vi "Main.vi"() -> ()   [LabVIEW 2018]
doc: "This example sets the RS-485 transceiver control modes for the specified port and performs a serial port read, a serial port write, or a combination of these actions. If all are selected, the VI will write the data first, read data and then close the VISA session that is opened to the port. This VI will wait until the specified number of bytes is received at the port or until a termination character is received. This example will work only with National Instruments RS-485 interfaces.\n\nThis example demonstrates the transceiver control modes available when using a National Instruments RS-485 product. When connecting one or several devices via RS-485, a user may want to cut down on the amount of wiring. Alternatively, some devices offer a certain wiring configuration that you may need to match. Determine the wiring needs of the connected serial device to determine which NI RS-485 transceiver control mode to choose.\n\nWhen you are communicating with a two-wire device, National Instruments recommends that you use the two-wire Auto Control mode. This mode handles the transmitter/receiver enabling for a two-wire connection in your hardware, so it reduces the software overhead required to perform this operation in your application program."
uses:
  estados.ctl
  mensagemFila.ctl
  <vilib>/Instr/_visa.llb/VISA Configure Serial Port (Instr).vi
panel:
  out "elements":T1[](array[typedef])
  out "# elements in queue":i32
  out "?":T2
  in  "Power":bool
  in  "flow control":u16(ring) caption="Ring" items=["None"=0, "XON/XOFF"=1, "RTS/CTS"=2, "DTR/DSR"=4]
  in  "stop bits":u16(ring)=10 caption="Ring" items=["1.0"=10, "1.5"=15, "2.0"=20]
  in  "parity":u16(ring) caption="Ring" items=["None", "Odd", "Even", "Mark", "Space"]
  in  "data bits":u16=8 caption="Numeric"
  in  "baud rate":u32=115200 caption="Numeric"
  out "SP = VP\nEscravo 2":bool
  out "SP = VP\nEscravo 1":bool
  out "Waveform Chart":T3(graph)
  in  "Sensor Escravo 2":u16(ring) caption="Ring" items=["LM35", "4 - 20 mA"]
  in  "Sensor Escravo 1":u16(ring) caption="Ring" items=["LM35", "4 - 20 mA"]
  in  "Verifica Sensor sl2":bool caption="Verifica Sensor\nEscravo 2"
  in  "Verifica Sensor sl1":bool caption="Verifica Sensor\nEscravo 1"
  in  "Envia Sensor sl2":bool caption="Seta Sensor\nEscravo 2"
  in  "Envia Sensor sl1":bool caption="Seta Sensor\nEscravo 1"
  out "Status":string caption="String"
  in  "Verifica SP sl2":bool caption="Verifica SP\nEscravo 2"
  in  "Verifica SP sl1":bool caption="Verifica SP\nEscravo 1"
  in  "SP escravo 2":u16 caption="SP Escravo 2"
  in  "Envia SP sl2":bool caption="Seta SP\nEscravo 2"
  in  "Envia SP sl1":bool caption="Seta SP\nEscravo 1"
  in  "SP escravo 1":u16 caption="SP Escravo 1"
  in  "VISA resource name":refnum<visa-resource-name>
  in  "stop":bool
  in  "dado":u16=4
  in  "opcode":u8=4 format="%.0b"
  in  "addr":u8=4 format="%.0x"
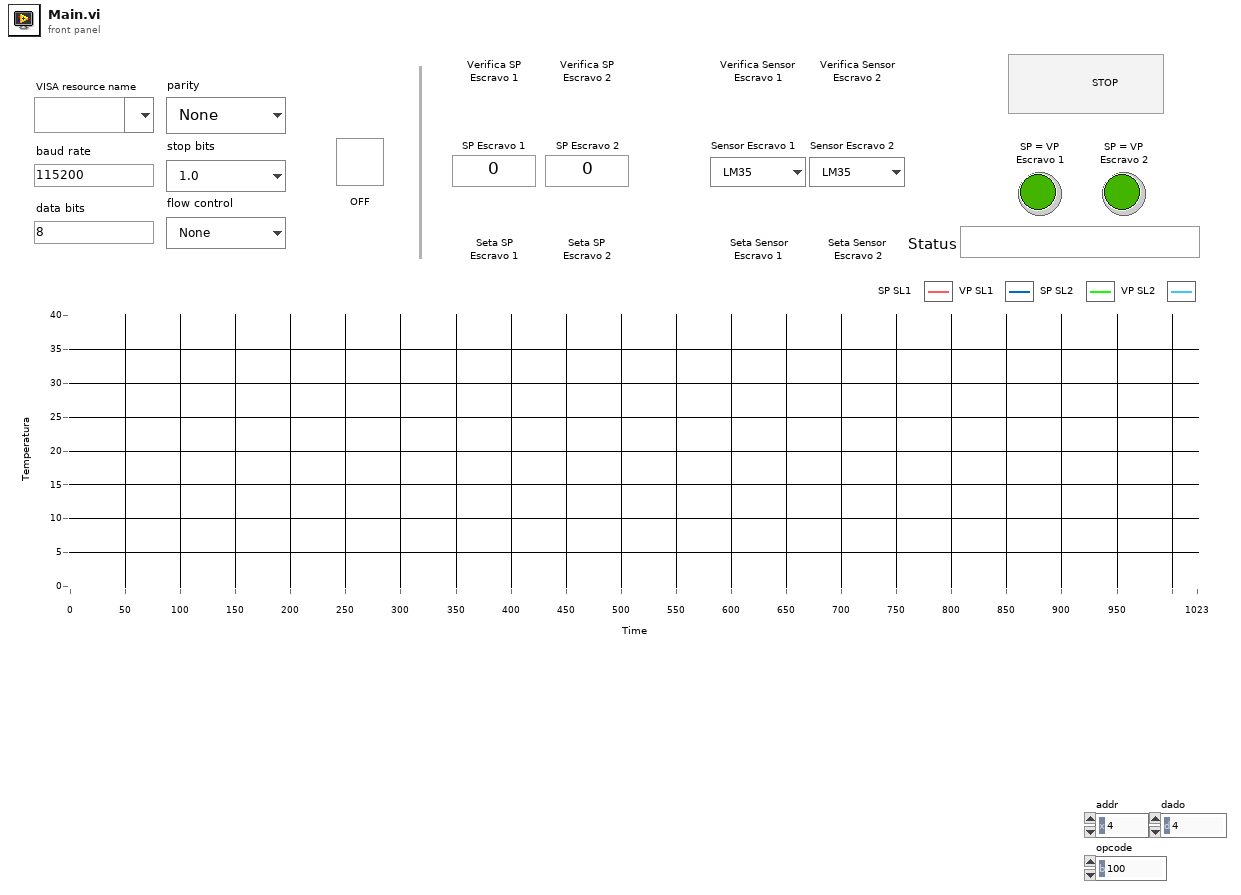
[diagram p1: front panel]
types:
  T1 = typedef "mensagemFila.ctl" = cluster{"Estado":T2, "Próximo Estado":T2, "Comando":string}
  T2 = typedef "estados.ctl" = enum16{"Idle", "Inicializa conexão", "Monta comando", "Envia comando", "Recebe resposta 1 escravo", "Recebe resposta 2 escravos", "Trata respostas", "Trata respostas 2 Escravos", "Encerra conexão", "Erro", "Stop", "Atualiza UI"}
  T3 = cluster{"plot 0":dbl, "plot 1":dbl, "plot 2":dbl, "plot 3":dbl}
  T4 = cluster{"SP escravo 1":refnum<vi>, "SP escravo 2":refnum<vi>, "Sensor Escravo 1":refnum<vi>, "Sensor Escravo 2":refnum<vi>, "SP = VP\nEscravo 1":refnum<vi>, "SP = VP\nEscravo 2":refnum<vi>, "Waveform Chart":refnum<vi>}
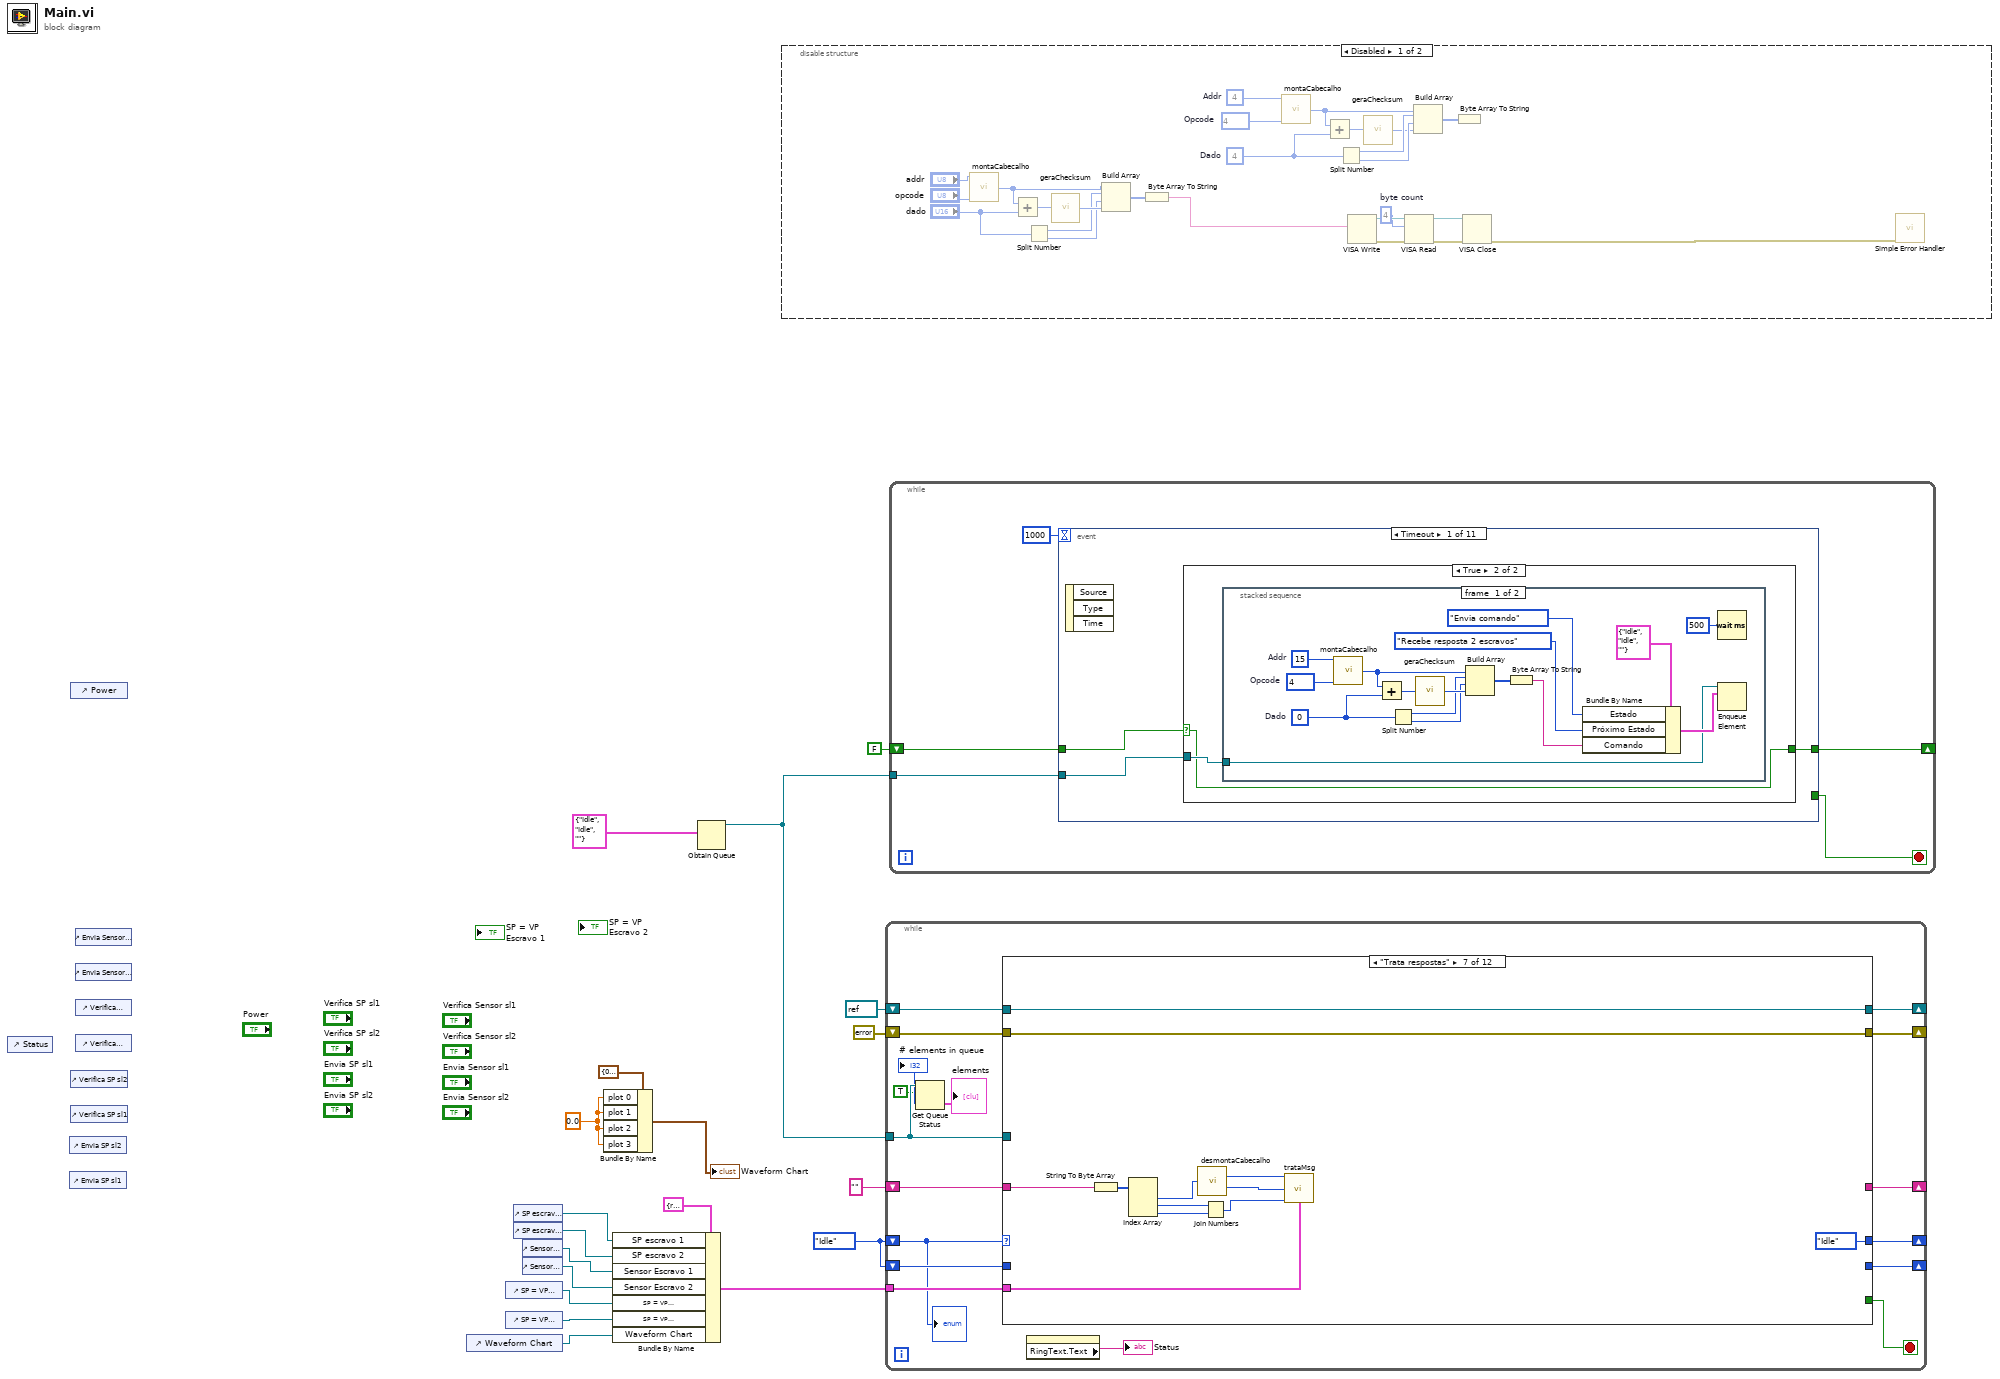
[diagram p0: block diagram]
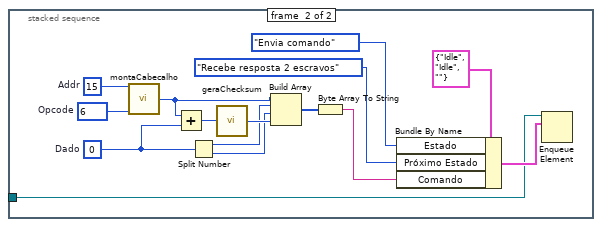
[diagram p4: hidden frame]
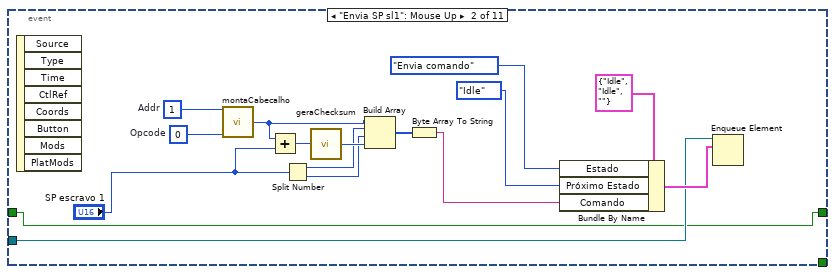
[diagram p5: hidden frame]
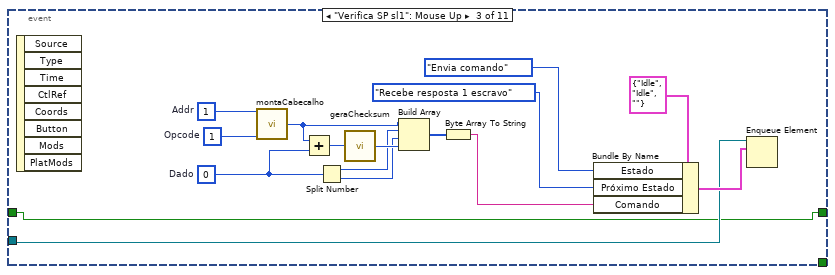
[diagram p6: hidden frame]
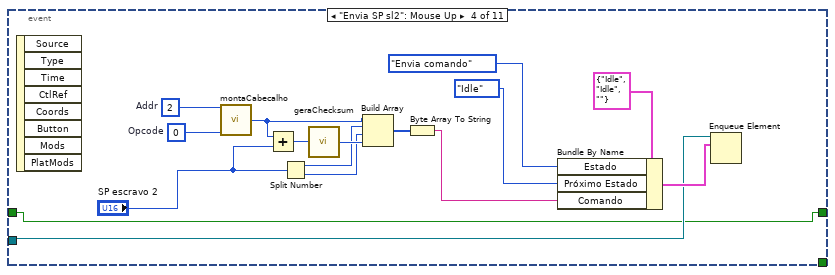
[diagram p7: hidden frame]
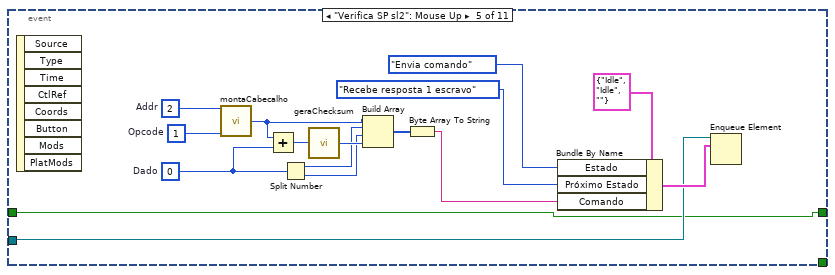
[diagram p8: hidden frame]
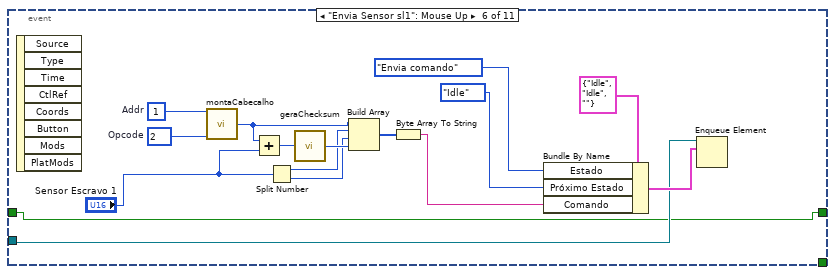
[diagram p9: hidden frame]
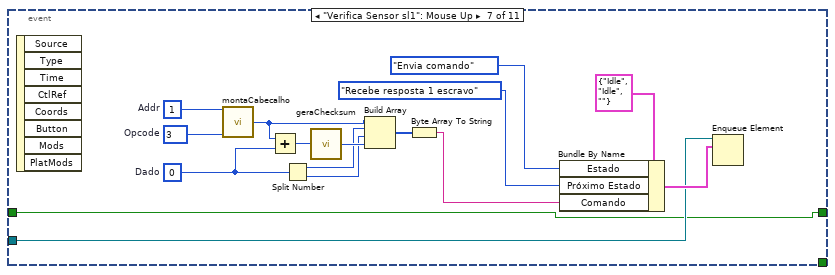
[diagram p10: hidden frame]
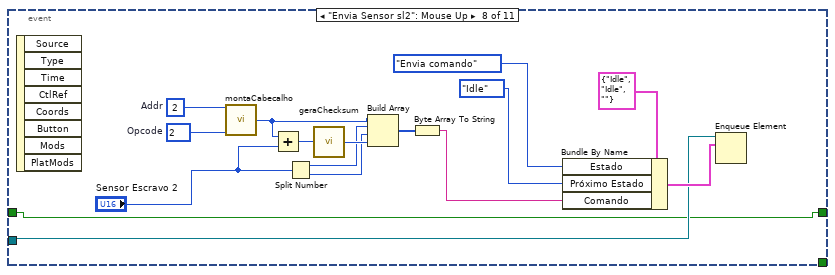
[diagram p11: hidden frame]
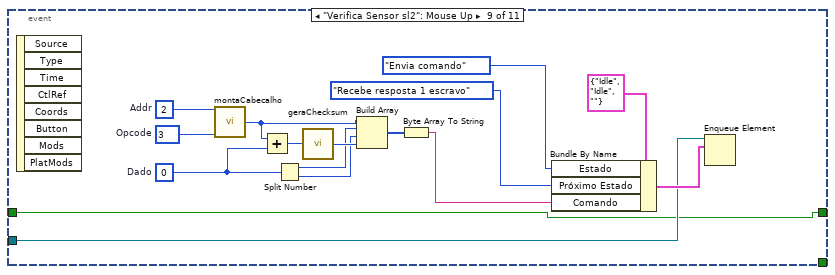
[diagram p12: hidden frame]
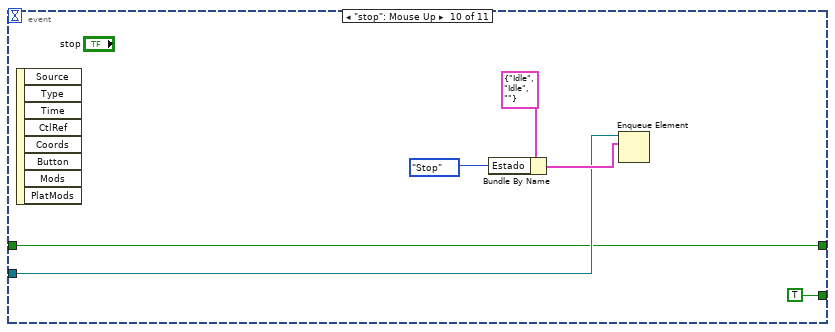
[diagram p13: hidden frame]
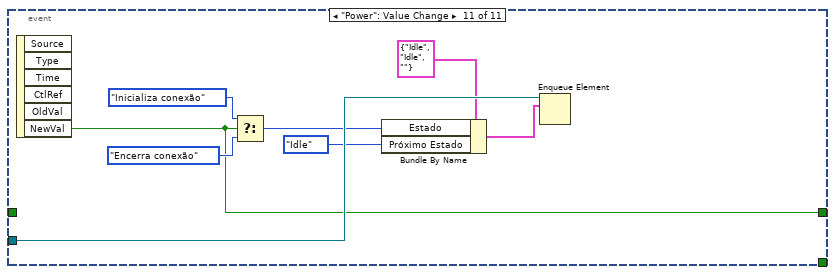
[diagram p14: hidden frame]
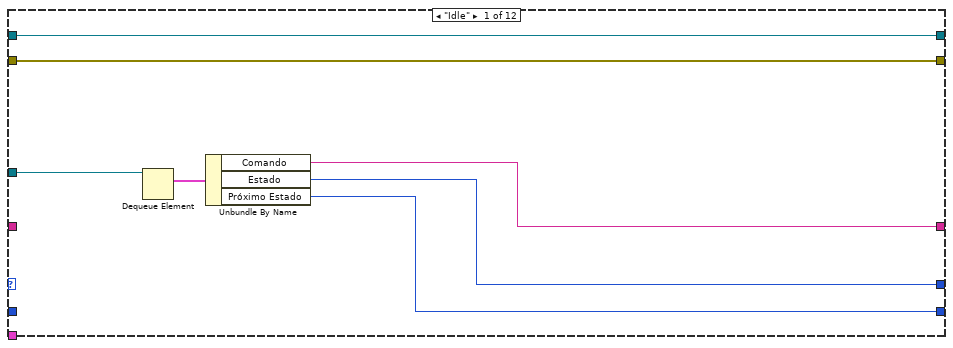
[diagram p15: hidden frame]
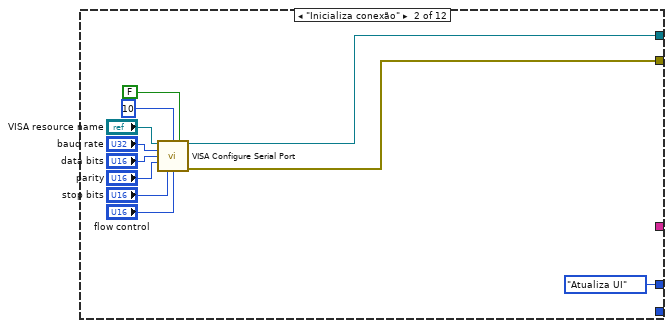
[diagram p16: hidden frame]
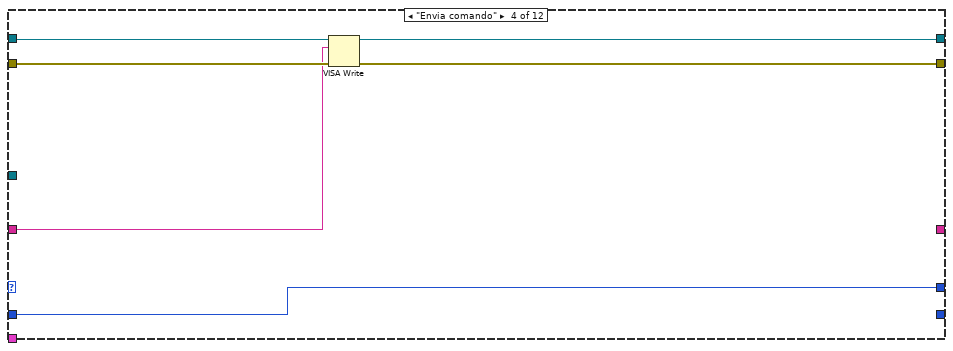
[diagram p18: hidden frame]
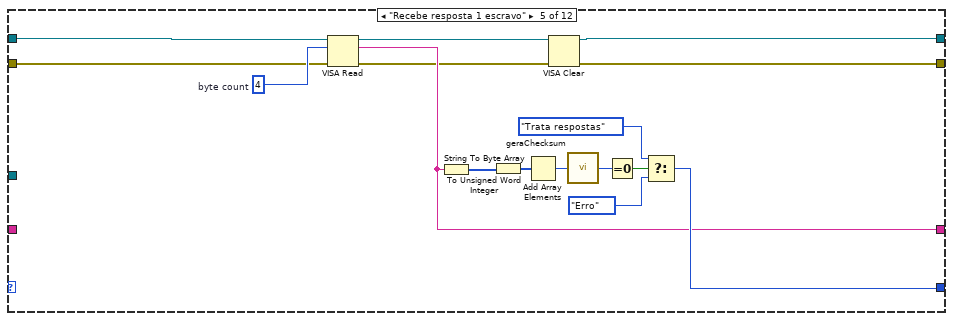
[diagram p19: hidden frame]
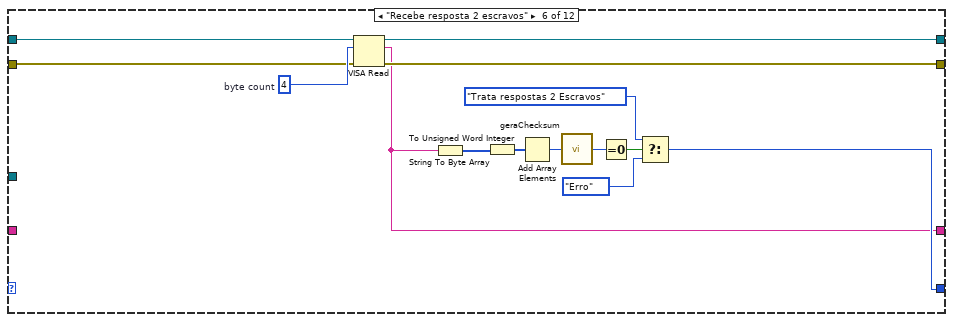
[diagram p20: hidden frame]
diagram:
  w2 = 0.0 ("element")
  w1 = estados."Idle"
  n1 = control-ref of="Status"() -> ()  [unwired: 1 out]
  n2 = control-ref of="Envia SP sl2"() -> ()  [unwired: 1 out]
  n3 = control-ref of="Envia SP sl1"() -> ()  [unwired: 1 out]
  n4 = control-ref of="Power"() -> ()  [unwired: 1 out]
  n5 = control-ref of="Verifica SP sl2"() -> ()  [unwired: 1 out]
  n6 = control-ref of="Verifica SP sl1"() -> ()  [unwired: 1 out]
  n7 = control-ref of="Envia Sensor sl2"() -> ()  [unwired: 1 out]
  n8 = control-ref of="Envia Sensor sl1"() -> ()  [unwired: 1 out]
  n9 = control-ref of="Verifica Sensor sl2"() -> ()  [unwired: 1 out]
  n10 = control-ref of="Verifica Sensor sl1"() -> ()  [unwired: 1 out]
  n11 = control-ref of="Waveform Chart"() -> (w6:refnum<vi>)
  n12 = control-ref of="SP = VP\nEscravo 1"() -> (w8:refnum<vi>)
  n13 = control-ref of="SP = VP\nEscravo 2"() -> (w7:refnum<vi>)
  n14 = control-ref of="SP escravo 1"() -> (w12:refnum<vi>)
  n15 = control-ref of="SP escravo 2"() -> (w11:refnum<vi>)
  n16 = control-ref of="Sensor Escravo 1"() -> (w10:refnum<vi>)
  n17 = control-ref of="Sensor Escravo 2"() -> (w9:refnum<vi>)
  n18 = Bundle By Name(cluster=T3 {"plot 0"=0.0, "plot 1"=0.0, "plot 2"=0.0, "plot 3"=0.0} ("input cluster"), "plot 0"=w2, "plot 1"=w2, "plot 2"=w2, "plot 3"=w2) -> (→"Waveform Chart":T3)
  n19 = Bundle By Name(cluster=T4 {"SP escravo 1"=refnum, "SP escravo 2"=refnum, "Sensor Escravo 1"=refnum, "Sensor Escravo 2"=refnum, "SP = VP\nEscravo 1"=refnum, "SP = VP\nEscravo 2"=refnum, "Waveform Chart"=refnum}, "SP escravo 1"=w12, "SP escravo 2"=w11, "Sensor Escravo 1"=w10, "Sensor Escravo 2"=w9, "SP = VP\nEscravo 1"=w8, "SP = VP\nEscravo 2"=w7, "Waveform Chart"=w6) -> (w5:T4)
  n20 = Obtain Queue(element data type=T1 {"Estado"=enum."Idle", "Próximo Estado"=enum."Idle", "Comando"=""}) -> (queue out=w16:refnum<queue>)  [unwired: 4 in, 2 out]
  n21 = disable-structure shown="Disabled" {
    frame Disabled {
      w26 = u8 4  # Addr
      w27 = u8 4  # Opcode
      w23 = u16 4  # Dado
      w39 = u32 4  # byte count
      n22 = call "montaCabecalho.vi"("addr"="addr", "opcode"="opcode") -> ("Cabeçalho"=w30:u8)  [unwired: 13 in]
      n23 = Add(x=w30, y="dado") -> (x+y=w36:u16)
      n24 = Split Number(x="dado") -> (hi(x)=w34:u8, lo(x)=w33:u8)
      n25 = call "geraChecksum.vi"("Soma"=w36) -> ("checksum"=w38:u8)  [unwired: 14 in]
      n26 = Build Array(w30, w34, w33, w38) -> (w37:u8[])
      n27 = Byte Array To String(unsigned byte array=w37) -> (string=w29:string)
      n28 = call "montaCabecalho.vi"("addr"=w26, "opcode"=w27) -> ("Cabeçalho"=w28:u8)  [unwired: 13 in]
      n29 = Add(x=w28, y=w23) -> (x+y=w22:u16)
      n30 = Split Number(x=w23) -> (hi(x)=w24:u8, lo(x)=w25:u8)
      n31 = VISA Write(write buffer=w29) -> (VISA resource name out=w44:refnum<visa-resource-name>, error out=w41:errorcluster)  [unwired: 2 in, 1 out]
      n32 = call "geraChecksum.vi"("Soma"=w22) -> ("checksum"=w20:u8)  [unwired: 14 in]
      n33 = VISA Read(VISA resource name=w44, byte count=w39, error in (no error)=w41) -> (VISA resource name out=w42:refnum<visa-resource-name>, error out=w43:errorcluster)  [unwired: 2 out]
      n34 = Build Array(w28, w24, w25, w20) -> (w21:u8[])
      n35 = Byte Array To String(unsigned byte array=w21) -> ()  [unwired: 1 out]
      n36 = VISA Close(VISA resource name=w42, error in (no error)=w43) -> (error out=w40:errorcluster)
      n37 = call <vilib>:"Simple Error Handler.vi"("error in (no error)"=w40) -> ()  [unwired: 1 in, 8 out]
    }
    frame Enabled {
    }
  }
  n38 = while {
    shift-right: [w59] -> _
    shift-left: w1 -> [w50]
    shift-right: [w58] -> _
    shift-left: errorcluster {"status"=FALSE, "code"=0, "source"=""} ("error out") -> [w60]
    shift-right: [w57] -> _
    shift-left: refnum<visa-resource-name> refnum ("VISA resource name out") -> [w61]
    shift-right: [w54] -> _
    shift-left: "" ("Dado") -> [w56]
    tunnel: w16 -> [w48]
    shift-right: [w52] -> _
    shift-left: w1 -> [w53]
    tunnel: w5 -> [w51]
    stop <- w55 stop-if-true
    n39 = Get Queue Status(queue=w48, return elements? (F)=TRUE) -> (# elements in queue=→"# elements in queue":i32, elements=→"elements":T1[])  [unwired: 1 in, 6 out]
    n40 = case shown="\"Trata respostas\"" w50 {
      tunnel: w61 -> [w67 _ w81 w87 w89 w117 w123 w140 w144 w146 w149 w155]
      tunnel: w60 -> [w68 _ w82 w88 w103 w116 w124 w141 w145 w147 w150 w154]
      tunnel: [w63 estados."Atualiza UI" _ w83 w95 w108 estados."Idle" estados."Recebe resposta 1 escravo" _ estados."Idle" _ estados."Idle"] -> w59
      tunnel: [w68 w71 w82 w85 w93 w115 w124 w141 w143 w147 w150 w154] -> w58
      tunnel: [w67 w70 w81 w86 w92 w114 w123 w140 _ w146 w149 w155] -> w57
      tunnel: w56 -> [_ _ w80 w84 _ _ w126 w132 _ _ _ _]
      tunnel: [_ _ _ _ _ _ _ _ _ _ TRUE _] -> w55
      tunnel: w48 -> [w66 _ _ _ _ _ _ _ _ _ w151 w156]
      tunnel: [w64 _ w80 _ w94 w105 _ _ _ _ _ _] -> w54
      tunnel: w53 -> [_ _ _ w83 _ _ _ _ _ _ _ _]
      tunnel: [w62 _ _ _ _ _ _ _ _ _ _ _] -> w52
      tunnel: w51 -> [_ _ _ _ _ _ w119 w131 _ _ _ _]
      frame "Idle" {
        n41 = Dequeue Element(queue=w66) -> (element=w65:T1)  [unwired: 2 in, 3 out]
        n42 = Unbundle By Name(w65) -> ("Comando"=w64:string, "Estado"=w63:T2, "Próximo Estado"=w62:T2)
      }
      frame "Inicializa conexão" {
        n43 = call-poly "VISA Configure Serial Port"("VISA resource name"="VISA resource name", "termination char\n(0xA = '\\n' = LF)"=u8 10 ("Termination Character"), "Enable Termination\nChar (T)"=FALSE ("End Read on Termination Character?"), "baud rate (9600)"="baud rate", "data bits (8)"="data bits", "parity (0:none)"="parity", "stop bits (10: 1 bit)"="stop bits", "flow control (0:none)"="flow control") -> ("VISA resource name out"=w70:refnum<visa-resource-name>, "error out"=w71:errorcluster)  [unwired: 2 in, 4 out]
      }
      frame "Monta comando" {
      }
      frame "Envia comando" {
        n44 = VISA Write(VISA resource name=w87, write buffer=w84, error in (no error)=w88) -> (VISA resource name out=w86:refnum<visa-resource-name>, error out=w85:errorcluster)  [unwired: 1 out]
      }
      frame "Recebe resposta 1 escravo" {
        w104 = u32 4  # byte count
        n45 = VISA Read(VISA resource name=w89, byte count=w104, error in (no error)=w103) -> (VISA resource name out=w90:refnum<visa-resource-name>, read buffer=w94:string, error out=w91:errorcluster)  [unwired: 1 out]
        n46 = String To Byte Array(string=w94) -> (unsigned byte array=w101:u8[])
        n47 = To Unsigned Word Integer(number=w101) -> (unsigned 16bit integer=w102:u16[])
        n48 = Add Array Elements(numeric array=w102) -> (sum=w100:u16)
        n49 = VISA Clear(VISA resource name=w90, error in (no error)=w91) -> (VISA resource name out=w92:refnum<visa-resource-name>, error out=w93:errorcluster)
        n50 = call "geraChecksum.vi"("Soma"=w100) -> ("checksum"=w99:u8)  [unwired: 14 in]
        n51 = Equal To 0?(x=w99) -> (x = 0?=w98:bool)
        n52 = Select(t=estados."Trata respostas", s=w98, f=estados."Erro") -> (s? t:f=w95:T2)
      }
      frame "Recebe resposta 2 escravos" {
        w118 = u32 4  # byte count
        n53 = VISA Read(VISA resource name=w117, byte count=w118, error in (no error)=w116) -> (VISA resource name out=w114:refnum<visa-resource-name>, read buffer=w105:string, error out=w115:errorcluster)  [unwired: 1 out]
        n54 = String To Byte Array(string=w105) -> (unsigned byte array=w112:u8[])
        n55 = To Unsigned Word Integer(number=w112) -> (unsigned 16bit integer=w113:u16[])
        n56 = Add Array Elements(numeric array=w113) -> (sum=w111:u16)
        n57 = call "geraChecksum.vi"("Soma"=w111) -> ("checksum"=w110:u8)  [unwired: 14 in]
        n58 = Equal To 0?(x=w110) -> (x = 0?=w109:bool)
        n59 = Select(t=estados."Trata respostas 2 Escravos", s=w109, f=estados."Erro") -> (s? t:f=w108:T2)
      }
      frame "Trata respostas" {
        n60 = String To Byte Array(string=w126) -> (unsigned byte array=w130:u8[])
        n61 = Index Array(array=w130) -> (element #1=w129:u8, element #2=w128:u8, element #3=w127:u8)  [unwired: 3 in]
        n62 = call "desmontaCabecalho.vi"("cabeçalho"=w129) -> ("addr"=w120:u8, "opcode"=w121:u8)  [unwired: 13 in]
        n63 = Join Numbers(hi=w128, lo=w127) -> ((hi.lo)=w122:u16)
        n64 = call "trataMsg.vi"("addr"=w120, "opcode"=w121, "dado"=w122, "ClusterUI"=w119) -> ()  [unwired: 12 in]
      }
      frame "Trata respostas 2 Escravos" {
        n65 = String To Byte Array(string=w132) -> (unsigned byte array=w139:u8[])
        n66 = Index Array(array=w139) -> (element #1=w138:u8, element #2=w137:u8, element #3=w136:u8)  [unwired: 3 in]
        n67 = call "desmontaCabecalho.vi"("cabeçalho"=w138) -> ("addr"=w133:u8, "opcode"=w134:u8)  [unwired: 13 in]
        n68 = Join Numbers(hi=w137, lo=w136) -> ((hi.lo)=w135:u16)
        n69 = call "trataMsg.vi"("addr"=w133, "opcode"=w134, "dado"=w135, "ClusterUI"=w131) -> ()  [unwired: 12 in]
      }
      frame "Encerra conexão" {
        n70 = VISA Close(VISA resource name=w144, error in (no error)=w145) -> (error out=w143:errorcluster)
      }
      frame "Erro" {
      }
      frame "Stop" {
        n71 = Release Queue(queue=w151) -> ()  [unwired: 2 in, 3 out]
      }
      frame "Atualiza UI" {
        n72 = stacked-sequence {
          tunnel: w156 -> [w170 w185]
          frame #0 {
            w162 = u8 15  # Addr
            w161 = u8 1  # Opcode
            w165 = u16 0  # Dado
            n73 = call "montaCabecalho.vi"("addr"=w162, "opcode"=w161) -> ("Cabeçalho"=w160:u8)  [unwired: 13 in]
            n74 = Add(x=w160, y=w165) -> (x+y=w166:u16)
            n75 = Split Number(x=w165) -> (hi(x)=w164:u8, lo(x)=w163:u8)
            n76 = call "geraChecksum.vi"("Soma"=w166) -> ("checksum"=w168:u8)  [unwired: 14 in]
            n77 = Build Array(w160, w164, w163, w168) -> (w167:u8[])
            n78 = Byte Array To String(unsigned byte array=w167) -> (string=w158:string)
            n79 = Bundle By Name(cluster=T1 {"Estado"=enum."Idle", "Próximo Estado"=enum."Idle", "Comando"=""}, "Estado"=estados."Envia comando", "Próximo Estado"=estados."Recebe resposta 2 escravos" ("Estado"), "Comando"=w158) -> (w171:T1)
            n80 = Enqueue Element(queue=w170, element=w171) -> ()  [unwired: 2 in, 3 out]
          }
          frame #1 {
            w177 = u8 15  # Addr
            w176 = u8 3  # Opcode
            w180 = u16 0  # Dado
            n81 = call "montaCabecalho.vi"("addr"=w177, "opcode"=w176) -> ("Cabeçalho"=w175:u8)  [unwired: 13 in]
            n82 = Add(x=w175, y=w180) -> (x+y=w181:u16)
            n83 = Split Number(x=w180) -> (hi(x)=w179:u8, lo(x)=w178:u8)
            n84 = call "geraChecksum.vi"("Soma"=w181) -> ("checksum"=w183:u8)  [unwired: 14 in]
            n85 = Build Array(w175, w179, w178, w183) -> (w182:u8[])
            n86 = Byte Array To String(unsigned byte array=w182) -> (string=w173:string)
            n87 = Bundle By Name(cluster=T1 {"Estado"=enum."Idle", "Próximo Estado"=enum."Idle", "Comando"=""}, "Estado"=estados."Envia comando", "Próximo Estado"=estados."Recebe resposta 2 escravos" ("Estado"), "Comando"=w173) -> (w186:T1)
            n88 = Enqueue Element(queue=w185, element=w186) -> ()  [unwired: 2 in, 3 out]
          }
        }
      }
    }
    n89 = property class="Enum (strict)"() -> ("RingText.Text"=→"Status":string)  [unwired: 2 in, 2 out]
    "?" <- w50
  }
  n90 = while {
    tunnel: w16 -> [w190]
    shift-right: [w188] -> _
    shift-left: FALSE ("NewVal") -> [w187]
    stop <- w191 stop-if-true
    n91 = event shown="[0] Timeout" {
      selector: _ -> [_ _ _ _ _ _ _ _ _ _ _]
      dyn-events: _ -> [_ _ _ _ _ _ _ _ _ _ _]
      timeout: 1000 -> [_ _ _ _ _ _ _ _ _ _ _]
      tunnel: [_ _ _ _ _ _ _ _ _ TRUE _] -> w191
      tunnel: w190 -> [w194 w231 w246 w263 w278 w295 w310 w327 w342 w358 w368]
      tunnel: [w192 w229 w245 w261 w277 w293 w309 w325 w341 w357 w363] -> w188
      tunnel: w187 -> [w193 w229 w245 w261 w277 w293 w309 w325 w341 w357 _]
      event Timeout {
        n92 = event-data() -> ()  [unwired: 1 in, 3 out]
        n93 = case shown="True" w193 {
          selector: w193 -> [w195 w196]
          tunnel: w194 -> [_ w197]
          tunnel: [w195 w196] -> w192
          frame False {
          }
          frame True {
            n94 = stacked-sequence {
              tunnel: w197 -> [w212 w227]
              frame #0 {
                w204 = u8 15  # Addr
                w203 = u8 4  # Opcode
                w207 = u16 0  # Dado
                n95 = call "montaCabecalho.vi"("addr"=w204, "opcode"=w203) -> ("Cabeçalho"=w202:u8)  [unwired: 13 in]
                n96 = Add(x=w202, y=w207) -> (x+y=w208:u16)
                n97 = Split Number(x=w207) -> (hi(x)=w206:u8, lo(x)=w205:u8)
                n98 = call "geraChecksum.vi"("Soma"=w208) -> ("checksum"=w210:u8)  [unwired: 14 in]
                n99 = Build Array(w202, w206, w205, w210) -> (w209:u8[])
                n100 = Byte Array To String(unsigned byte array=w209) -> (string=w200:string)
                n101 = Bundle By Name(cluster=T1 {"Estado"=enum."Idle", "Próximo Estado"=enum."Idle", "Comando"=""}, "Estado"=estados."Envia comando", "Próximo Estado"=estados."Recebe resposta 2 escravos" ("Estado"), "Comando"=w200) -> (w213:T1)
                n102 = Wait (ms)(milliseconds to wait=u32 500) -> ()  [unwired: 1 out]
                n103 = Enqueue Element(queue=w212, element=w213) -> ()  [unwired: 2 in, 3 out]
              }
              frame #1 {
                w219 = u8 15  # Addr
                w218 = u8 6  # Opcode
                w222 = u16 0  # Dado
                n104 = call "montaCabecalho.vi"("addr"=w219, "opcode"=w218) -> ("Cabeçalho"=w217:u8)  [unwired: 13 in]
                n105 = Add(x=w217, y=w222) -> (x+y=w223:u16)
                n106 = Split Number(x=w222) -> (hi(x)=w221:u8, lo(x)=w220:u8)
                n107 = call "geraChecksum.vi"("Soma"=w223) -> ("checksum"=w225:u8)  [unwired: 14 in]
                n108 = Build Array(w217, w221, w220, w225) -> (w224:u8[])
                n109 = Byte Array To String(unsigned byte array=w224) -> (string=w215:string)
                n110 = Bundle By Name(cluster=T1 {"Estado"=enum."Idle", "Próximo Estado"=enum."Idle", "Comando"=""}, "Estado"=estados."Envia comando", "Próximo Estado"=estados."Recebe resposta 2 escravos" ("Estado"), "Comando"=w215) -> (w228:T1)
                n111 = Enqueue Element(queue=w227, element=w228) -> ()  [unwired: 2 in, 3 out]
              }
            }
          }
        }
      }
      event "Envia SP sl1": Mouse Up {
        w237 = u8 1  # Addr
        w236 = u8 0  # Opcode
        n112 = event-data() -> ()  [unwired: 1 in, 8 out]
        n113 = call "montaCabecalho.vi"("addr"=w237, "opcode"=w236) -> ("Cabeçalho"=w235:u8)  [unwired: 13 in]
        n114 = Add(x=w235, y="SP escravo 1") -> (x+y=w240:u16)
        n115 = Split Number(x="SP escravo 1") -> (hi(x)=w239:u8, lo(x)=w238:u8)
        n116 = call "geraChecksum.vi"("Soma"=w240) -> ("checksum"=w242:u8)  [unwired: 14 in]
        n117 = Build Array(w235, w239, w238, w242) -> (w241:u8[])
        n118 = Byte Array To String(unsigned byte array=w241) -> (string=w233:string)
        n119 = Bundle By Name(cluster=T1 {"Estado"=enum."Idle", "Próximo Estado"=enum."Idle", "Comando"=""}, "Estado"=estados."Envia comando", "Próximo Estado"=estados."Idle" ("Estado"), "Comando"=w233) -> (w244:T1)
        n120 = Enqueue Element(queue=w231, element=w244) -> ()  [unwired: 2 in, 3 out]
      }
      event "Verifica SP sl1": Mouse Up {
        w252 = u8 1  # Addr
        w251 = u8 1  # Opcode
        w255 = u16 0  # Dado
        n121 = event-data() -> ()  [unwired: 1 in, 8 out]
        n122 = call "montaCabecalho.vi"("addr"=w252, "opcode"=w251) -> ("Cabeçalho"=w250:u8)  [unwired: 13 in]
        n123 = Add(x=w250, y=w255) -> (x+y=w256:u16)
        n124 = Split Number(x=w255) -> (hi(x)=w254:u8, lo(x)=w253:u8)
        n125 = call "geraChecksum.vi"("Soma"=w256) -> ("checksum"=w258:u8)  [unwired: 14 in]
        n126 = Build Array(w250, w254, w253, w258) -> (w257:u8[])
        n127 = Byte Array To String(unsigned byte array=w257) -> (string=w248:string)
        n128 = Bundle By Name(cluster=T1 {"Estado"=enum."Idle", "Próximo Estado"=enum."Idle", "Comando"=""}, "Estado"=estados."Envia comando", "Próximo Estado"=estados."Recebe resposta 1 escravo" ("Estado"), "Comando"=w248) -> (w260:T1)
        n129 = Enqueue Element(queue=w246, element=w260) -> ()  [unwired: 2 in, 3 out]
      }
      event "Envia SP sl2": Mouse Up {
        w269 = u8 2  # Addr
        w268 = u8 0  # Opcode
        n130 = event-data() -> ()  [unwired: 1 in, 8 out]
        n131 = call "montaCabecalho.vi"("addr"=w269, "opcode"=w268) -> ("Cabeçalho"=w267:u8)  [unwired: 13 in]
        n132 = Add(x=w267, y="SP escravo 2") -> (x+y=w272:u16)
        n133 = Split Number(x="SP escravo 2") -> (hi(x)=w271:u8, lo(x)=w270:u8)
        n134 = call "geraChecksum.vi"("Soma"=w272) -> ("checksum"=w274:u8)  [unwired: 14 in]
        n135 = Build Array(w267, w271, w270, w274) -> (w273:u8[])
        n136 = Byte Array To String(unsigned byte array=w273) -> (string=w265:string)
        n137 = Bundle By Name(cluster=T1 {"Estado"=enum."Idle", "Próximo Estado"=enum."Idle", "Comando"=""}, "Estado"=estados."Envia comando", "Próximo Estado"=estados."Idle" ("Estado"), "Comando"=w265) -> (w276:T1)
        n138 = Enqueue Element(queue=w263, element=w276) -> ()  [unwired: 2 in, 3 out]
      }
      event "Verifica SP sl2": Mouse Up {
        w284 = u8 2  # Addr
        w283 = u8 1  # Opcode
        w287 = u16 0  # Dado
        n139 = event-data() -> ()  [unwired: 1 in, 8 out]
        n140 = call "montaCabecalho.vi"("addr"=w284, "opcode"=w283) -> ("Cabeçalho"=w282:u8)  [unwired: 13 in]
        n141 = Add(x=w282, y=w287) -> (x+y=w288:u16)
        n142 = Split Number(x=w287) -> (hi(x)=w286:u8, lo(x)=w285:u8)
        n143 = call "geraChecksum.vi"("Soma"=w288) -> ("checksum"=w290:u8)  [unwired: 14 in]
        n144 = Build Array(w282, w286, w285, w290) -> (w289:u8[])
        n145 = Byte Array To String(unsigned byte array=w289) -> (string=w280:string)
        n146 = Bundle By Name(cluster=T1 {"Estado"=enum."Idle", "Próximo Estado"=enum."Idle", "Comando"=""}, "Estado"=estados."Envia comando", "Próximo Estado"=estados."Recebe resposta 1 escravo" ("Estado"), "Comando"=w280) -> (w292:T1)
        n147 = Enqueue Element(queue=w278, element=w292) -> ()  [unwired: 2 in, 3 out]
      }
      event "Envia Sensor sl1": Mouse Up {
        w301 = u8 1  # Addr
        w300 = u8 2  # Opcode
        n148 = event-data() -> ()  [unwired: 1 in, 8 out]
        n149 = call "montaCabecalho.vi"("addr"=w301, "opcode"=w300) -> ("Cabeçalho"=w299:u8)  [unwired: 13 in]
        n150 = Add(x=w299, y="Sensor Escravo 1") -> (x+y=w304:u16)
        n151 = Split Number(x="Sensor Escravo 1") -> (hi(x)=w303:u8, lo(x)=w302:u8)
        n152 = call "geraChecksum.vi"("Soma"=w304) -> ("checksum"=w306:u8)  [unwired: 14 in]
        n153 = Build Array(w299, w303, w302, w306) -> (w305:u8[])
        n154 = Byte Array To String(unsigned byte array=w305) -> (string=w297:string)
        n155 = Bundle By Name(cluster=T1 {"Estado"=enum."Idle", "Próximo Estado"=enum."Idle", "Comando"=""}, "Estado"=estados."Envia comando", "Próximo Estado"=estados."Idle" ("Estado"), "Comando"=w297) -> (w308:T1)
        n156 = Enqueue Element(queue=w295, element=w308) -> ()  [unwired: 2 in, 3 out]
      }
      event "Verifica Sensor sl1": Mouse Up {
        w316 = u8 1  # Addr
        w315 = u8 3  # Opcode
        w319 = u16 0  # Dado
        n157 = event-data() -> ()  [unwired: 1 in, 8 out]
        n158 = call "montaCabecalho.vi"("addr"=w316, "opcode"=w315) -> ("Cabeçalho"=w314:u8)  [unwired: 13 in]
        n159 = Add(x=w314, y=w319) -> (x+y=w320:u16)
        n160 = Split Number(x=w319) -> (hi(x)=w318:u8, lo(x)=w317:u8)
        n161 = call "geraChecksum.vi"("Soma"=w320) -> ("checksum"=w322:u8)  [unwired: 14 in]
        n162 = Build Array(w314, w318, w317, w322) -> (w321:u8[])
        n163 = Byte Array To String(unsigned byte array=w321) -> (string=w312:string)
        n164 = Bundle By Name(cluster=T1 {"Estado"=enum."Idle", "Próximo Estado"=enum."Idle", "Comando"=""}, "Estado"=estados."Envia comando", "Próximo Estado"=estados."Recebe resposta 1 escravo" ("Estado"), "Comando"=w312) -> (w324:T1)
        n165 = Enqueue Element(queue=w310, element=w324) -> ()  [unwired: 2 in, 3 out]
      }
      event "Envia Sensor sl2": Mouse Up {
        w333 = u8 2  # Addr
        w332 = u8 2  # Opcode
        n166 = event-data() -> ()  [unwired: 1 in, 8 out]
        n167 = call "montaCabecalho.vi"("addr"=w333, "opcode"=w332) -> ("Cabeçalho"=w331:u8)  [unwired: 13 in]
        n168 = Add(x=w331, y="Sensor Escravo 2") -> (x+y=w336:u16)
        n169 = Split Number(x="Sensor Escravo 2") -> (hi(x)=w335:u8, lo(x)=w334:u8)
        n170 = call "geraChecksum.vi"("Soma"=w336) -> ("checksum"=w338:u8)  [unwired: 14 in]
        n171 = Build Array(w331, w335, w334, w338) -> (w337:u8[])
        n172 = Byte Array To String(unsigned byte array=w337) -> (string=w329:string)
        n173 = Bundle By Name(cluster=T1 {"Estado"=enum."Idle", "Próximo Estado"=enum."Idle", "Comando"=""}, "Estado"=estados."Envia comando", "Próximo Estado"=estados."Idle" ("Estado"), "Comando"=w329) -> (w340:T1)
        n174 = Enqueue Element(queue=w327, element=w340) -> ()  [unwired: 2 in, 3 out]
      }
      event "Verifica Sensor sl2": Mouse Up {
        w348 = u8 2  # Addr
        w347 = u8 3  # Opcode
        w346 = u16 0  # Dado
        n175 = event-data() -> ()  [unwired: 1 in, 8 out]
        n176 = call "montaCabecalho.vi"("addr"=w348, "opcode"=w347) -> ("Cabeçalho"=w350:u8)  [unwired: 13 in]
        n177 = Add(x=w350, y=w346) -> (x+y=w353:u16)
        n178 = Split Number(x=w346) -> (hi(x)=w352:u8, lo(x)=w351:u8)
        n179 = call "geraChecksum.vi"("Soma"=w353) -> ("checksum"=w355:u8)  [unwired: 14 in]
        n180 = Build Array(w350, w352, w351, w355) -> (w354:u8[])
        n181 = Byte Array To String(unsigned byte array=w354) -> (string=w349:string)
        n182 = Bundle By Name(cluster=T1 {"Estado"=enum."Idle", "Próximo Estado"=enum."Idle", "Comando"=""}, "Estado"=estados."Envia comando", "Próximo Estado"=estados."Recebe resposta 1 escravo" ("Estado"), "Comando"=w349) -> (w356:T1)
        n183 = Enqueue Element(queue=w342, element=w356) -> ()  [unwired: 2 in, 3 out]
      }
      event "stop": Mouse Up {
        n184 = event-data() -> ()  [unwired: 1 in, 8 out]
        n185 = Bundle By Name(cluster=T1 {"Estado"=enum."Idle", "Próximo Estado"=enum."Idle", "Comando"=""}, "Estado"=estados."Stop") -> (w361:T1)
        n186 = Enqueue Element(queue=w358, element=w361) -> ()  [unwired: 2 in, 3 out]
      }
      event "Power": Value Change {
        n187 = event-data() -> ("NewVal"=w363:bool)  [unwired: 1 in, 5 out]
        n188 = Select(t=estados."Inicializa conexão", s=w363, f=estados."Encerra conexão") -> (s? t:f=w367:T2)
        n189 = Bundle By Name(cluster=T1 {"Estado"=enum."Idle", "Próximo Estado"=enum."Idle", "Comando"=""}, "Estado"=w367, "Próximo Estado"=estados."Idle") -> (w365:T1)
        n190 = Enqueue Element(queue=w368, element=w365) -> ()  [unwired: 2 in, 3 out]
      }
    }
  }
